vi "_emi_Close Loop Array.vi"(5 "Loop IDs in":u16[](array[numeric]), 9 "error in (no error)":errorcluster) -> (10 "error out":errorcluster)   [LabVIEW 2010]
doc: "Destroy the Loop, should be performed after the outer loop exists in prepreation of program close.\n\nExecutes as normal on error"
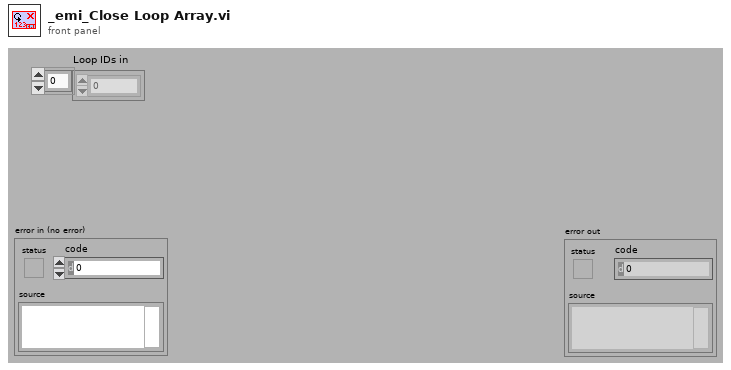
[diagram p1: front panel]
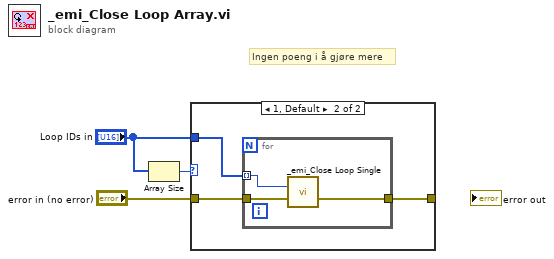
[diagram p0: block diagram]
diagram:
  # "Ingen poeng i å gjøre mere"
  n1 = Array Size(array="Loop IDs in") -> (size(s)=w2:i32)
  n2 = case shown="1, Default" w2 {
    tunnel: "error in (no error)" -> [w4 w7]
    tunnel: [w4 w6] -> _
    tunnel: "Loop IDs in" -> [_ w5]
    frame 0 {
    }
    frame 1, Default {
      n3 = for {
        tunnel: w7 -> [w10]
        tunnel: [w9] -> w6
        tunnel: w5 -> [w8] mode=indexing
        n4 = call "_emi_Close Loop Single.vi"("Loop ID in"=w8, "error in (no error)"=w10) -> ("error out"=w9:errorcluster)  [unwired: 13 in]
      }
    }
  }
